vi "Vision Processing.vi"(4 "error in (no error)":errorcluster) -> ()   [LabVIEW 2011]
uses:
  Robot Global Data.vi
  System Set Points and States.vi
  <vilib>/vision/NI_Vision_Development_Module.lvlib
panel:
  in  "lum max":sgl(slide) scale=0.0..255.0
  in  "lum min":sgl(slide) scale=0.0..255.0
  out "Enabled":bool
  out "Target Info":T1(array[cluster])
  in  "Area Size Limit":i32=444
  in  "Particle Count Limit":i32=8
  in  "Score Limits":T2={"Rect Coverage"=76.0, "Aspect Ratio"=70.0, "X Edge Strength"=40.0, "Y Edge Strength"=60.0}
  out "Processed Image":T3(plugin-control)
  # "Instructions:\nProcessing the reflective tape that is illuminated by a ring light can be based\non color or light intensity.\nParticles within the image are scored by rectangle coverage, aspect ratio, and\nfor being hollow with a bold edge. A particle is considered a target if all scores\nare above the score limits. Particles can be annotated -- surrounded by\na rectangle and scores drawn to the left .\nTo control the number of particles being scored, use the count limit and the size\nlimit."
  # "To debug, Enable using the View button.\nFor color processing, you can click in the image to select the color for processing."
  # "Enable by clicking the View button.\nGreen scores are above the limit, orange are below. Inner/outer rect\nindicates all passed."
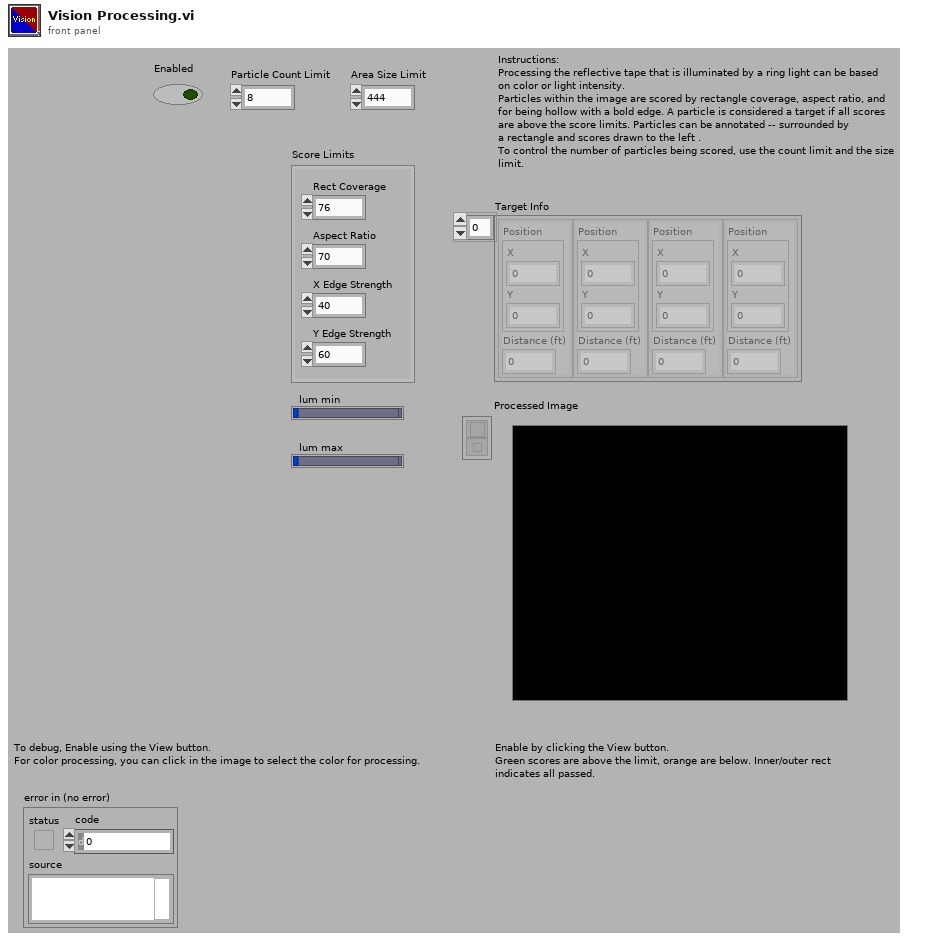
[diagram p1: front panel]
types:
  T1 = cluster{"Position":cluster{"X":dbl, "Y":dbl}, "Distance (ft)":dbl}[]
  T2 = cluster{"Rect Coverage":dbl, "Aspect Ratio":dbl, "X Edge Strength":dbl, "Y Edge Strength":dbl}
  T3 = typedef "IMAQ Image.ctl" = refnum<image>
  T4 = typedef "Image Type" = u32
  T5 = typedef "WPI_CameraDevRef.ctl" = cluster{"Camera Address":string, "CameraStatus":errorcluster, "Acquire Image Notifier":refnum<notifier>}
  T6 = typedef "WPI_CameraImageSize.ctl" = enum16{"640x480", "320x240", "160x120"}
  T7 = cluster{cluster{"Left":dbl, "Top":dbl, "Right":dbl, "Bottom":dbl}, dbl[]}[]
  T8 = cluster{"Left":dbl, "Top":dbl, "Right":dbl, "Bottom":dbl}
  T9 = cluster{"Target Center (-1 to 1)":cluster{"X":dbl, "Y":dbl}, "Distance (ft)":dbl}
  T10 = cluster{"Target Center (-1 to 1)":cluster{"X":dbl, "Y":dbl}, "Distance (ft)":dbl}[]
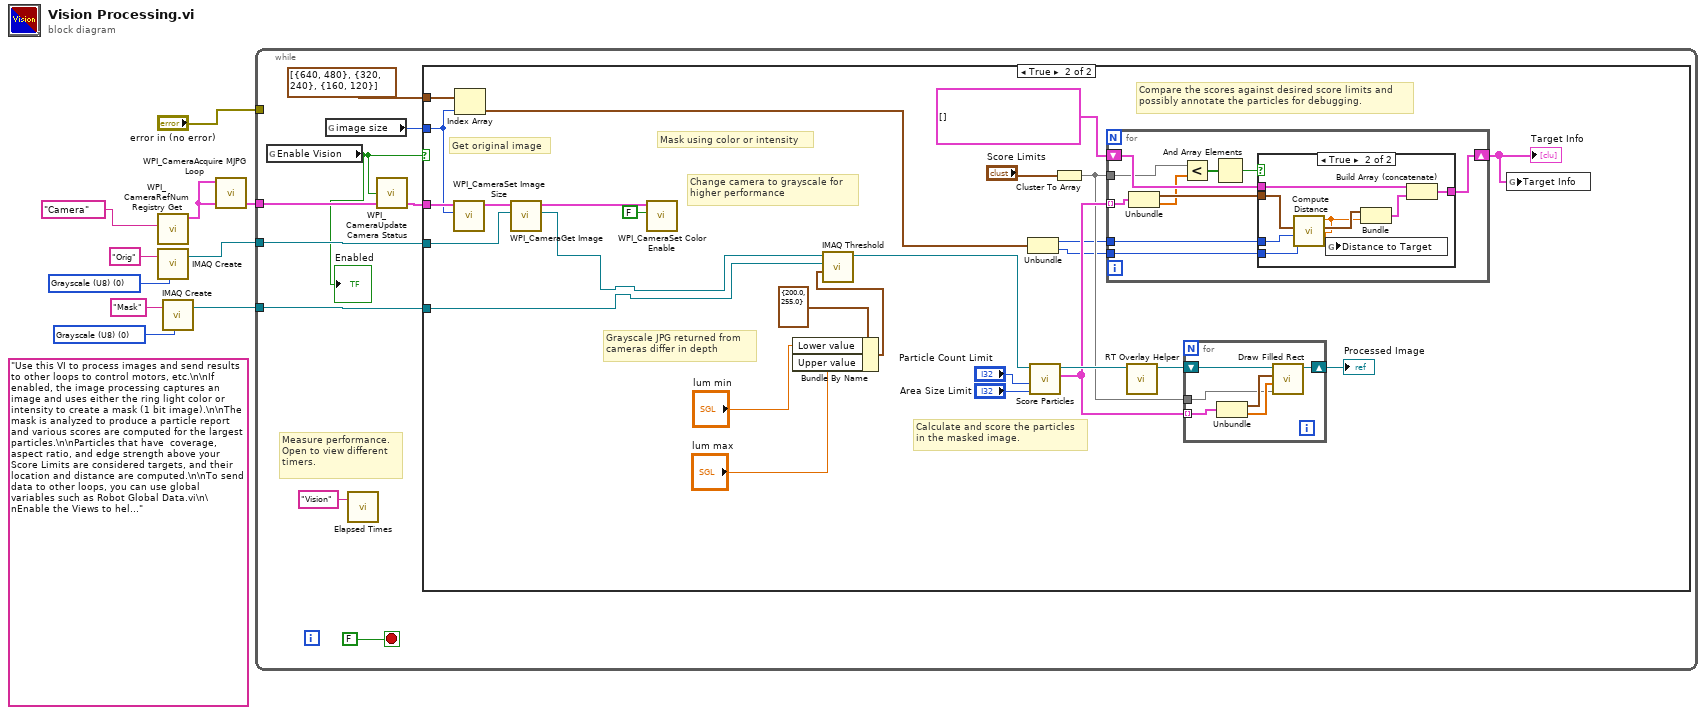
[diagram p0: block diagram]
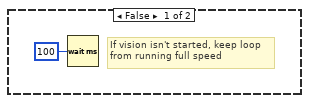
[diagram p2: hidden frame]
diagram:
  w3 = T4 0 items=["Grayscale (U8)", "Grayscale (I16)", "Grayscale (SGL)", "Complex (CSG)", "RGB (U32)", "HSL (U32)", "RGB (U64)", "Grayscale (U16)"] ("Image Type")
  (unwired) "Use this VI to process images and send results to other loops to control motors, etc.\n\nIf enabled, the image processing captures an image and uses either the ring light color or intensity to create a mask (1 bit image).\n\nThe mask is analyzed to produce a particle report and various scores are computed for the largest particles.\n\nParticles that have  coverage, aspect ratio, and edge strength above your Score Limits are considered targets, and their location and distance are computed.\n\nTo send data to other loops, you can use global variables such as Robot Global Data.vi\n\nEnable the Views to help debug color settings. Disable the View to speed up processing."
  w8 = T4 0 items=["Grayscale (U8)", "Grayscale (I16)", "Grayscale (SGL)", "Complex (CSG)", "RGB (U32)", "HSL (U32)", "RGB (U64)", "Grayscale (U16)"] ("Image Type")
  n1 = call <vilib>:"WPI_CameraRefNum Registry Get.vi"("refnum name"="Camera") -> ("CameraDevRef"=w6:T5)  [unwired: 9 in, 1 out]
  n2 = call "IMAQ Create"("Image Name"="Orig", "Image Type"=w8) -> ("New Image"=w7:T3)  [unwired: 2 in, 2 out]
  n3 = call "IMAQ Create"("Image Name"="Mask", "Image Type"=w3) -> ("New Image"=w2:T3)  [unwired: 2 in, 2 out]
  n4 = call <vilib>:"WPI_CameraAcquire MJPG Loop.vi"("CameraDevRef"=w6) -> ()  [unwired: 11 in]
  n5 = while {
    tunnel: w7 -> [w17]
    tunnel: w6 -> [w16]
    tunnel: "error in (no error)" -> [_]
    tunnel: w2 -> [w11]
    stop <- FALSE stop-if-true
    # "Measure performance.\nOpen to view different\ntimers."
    n6 = global read "Robot Global Data.vi" "Enable Vision"() -> (w10:bool)
    "Enabled" <- w10
    n7 = global read "Robot Global Data.vi" "image size"() -> (w13:T6)
    n8 = call "Elapsed Times.vi"("Call Name"="Vision") -> ()  [unwired: 2 in, 1 out]
    n9 = call <vilib>:"WPI_CameraUpdate Camera Status.vi"("CameraDevRef In"=w16, "Enable Vision"=w10) -> ("CameraDevRef Out"=w15:T5)  [unwired: 3 in]
    n10 = case shown="True" w10 {
      tunnel: w17 -> [_ w39]
      tunnel: w15 -> [_ w35]
      tunnel: w13 -> [_ w33]
      tunnel: cluster{i32, i32}[] [{640, 480}, {320, 240}, {160, 120}] -> [_ w32]
      tunnel: w11 -> [_ w23]
      frame False {
        # "If vision isn't started, keep loop\nfrom running full speed"
        n11 = Wait (ms)(milliseconds to wait=u32 100) -> ()  [unwired: 1 out]
      }
      frame True {
        # "Grayscale JPG returned from\ncameras differ in depth"
        # "Change camera to grayscale for\nhigher performance"
        # "Compare the scores against desired score limits and\npossibly annotate the particles for debugging."
        # "Calculate and score the particles\nin the masked image."
        # "Mask using color or intensity"
        # "Get original image"
        n12 = call <vilib>:"WPI_CameraSet Image Size.vi"("Image Size"=w33, "CameraDevRef"=w35) -> ("CameraDevRef Out"=w36:T5)  [unwired: 8 in, 1 out]
        n13 = Index Array(array=w32, index=w33) -> (element=w29:cluster{i32, i32})
        n14 = call <vilib>:"WPI_CameraGet Image.vi"("Image"=w39, "CameraDevRef"=w36) -> ("Image Out"=w22:T3, "CameraDevRef Out"=w38:T5)  [unwired: 7 in, 1 out]
        n15 = call <vilib>:"WPI_CameraSet Color Enable.vi"("Color Enabled"=FALSE, "CameraDevRef"=w38) -> ()  [unwired: 8 in, 2 out]
        n16 = Bundle By Name(cluster=cluster{"Lower value":sgl, "Upper value":sgl} {"Lower value"=200.0, "Upper value"=255.0} ("Range"), "Lower value"="lum min", "Upper value"="lum max") -> (w24:cluster{"Lower value":sgl, "Upper value":sgl})
        n17 = call "IMAQ Threshold"("Range"=w24, "Image Dst"=w23, "Image Src"=w22) -> ("Image Dst Out"=w34:T3)  [unwired: 3 in, 5 out]
        n18 = Unbundle(w29) -> (w31:i32, w30:i32)
        n19 = call "Score Particles.vi"("Area Size Limit"="Area Size Limit", "Particle Count Limit"="Particle Count Limit", "Image Refnum in"=w34) -> ("Scored Particle Info"=w43:T7, "Image Refnum out"=w46:T3)  [unwired: 7 in]
        n20 = Cluster To Array(cluster="Score Limits") -> (array=w42:dbl[])
        n21 = for {
          shift-right: [w61] -> w37
          shift-left: T1 [] -> [w62]
          tunnel: w31 -> [w60]
          tunnel: w43 -> [w58] mode=indexing
          tunnel: w42 -> [w54]
          tunnel: w30 -> [w53]
          n22 = Unbundle(w58) -> (w59:T8, w55:dbl[])
          n23 = Less?(x=w54, y=w55) -> (x < y?=w57:bool[])
          n24 = And Array Elements(Boolean array=w57) -> (logical AND=w56:bool)
          n25 = case shown="True" w56 {
            tunnel: w62 -> [w63 w71]
            tunnel: [w63 w70] -> w61
            tunnel: w59 -> [_ w67]
            tunnel: w60 -> [_ w68]
            tunnel: w53 -> [_ w66]
            frame False {
            }
            frame True {
              n26 = call "Compute Distance.vi"("Y Image Resolution"=w66, "X Image Resolution"=w68, "Bounding Box"=w67) -> ("Target Center (-1 to 1)"=w65:cluster{"X":dbl, "Y":dbl}, "Distance (ft)"=w64:dbl)  [unwired: 7 in]
              n27 = global write "System Set Points and States.vi" "Distance to Target"(w64) -> ()
              n28 = Bundle("Target Center (-1 to 1)"=w65, "Distance (ft)"=w64) -> (w69:T9)  [unwired: 1 in]
              n29 = Build Array (concatenate)(w71, w69) -> (w70:T10)
            }
          }
        }
        "Target Info" <- w37
        n30 = call "RT Overlay Helper.vi"("Refnum in"=w46) -> ("Refnum out"=w27:T3)  [unwired: 10 in]
        n31 = for {
          shift-right: [w51] -> w26
          shift-left: w27 -> [w52]
          tunnel: w43 -> [w48] mode=indexing
          tunnel: w42 -> [w47]
          n32 = Unbundle(w48) -> (w49:T8, w50:dbl[])
          n33 = call "Draw Filled Rect.vi"("Limits"=w47, "Scores"=w50, "Bounding Box"=w49, "image in"=w52) -> ("image out"=w51:T3)  [unwired: 7 in]
        }
        "Processed Image" <- w26
        n34 = global write "Robot Global Data.vi" "Target Info"(w37) -> ()
      }
    }
  }
